vi "CRYGet Graph Name From Graph Type.vi"(11 "Graph Type":string) -> (2 "Type":enum16{"Curves", "Values", "Results", "WFM"}(ring), 3 "Graph Name":string)   [LabVIEW 2013]
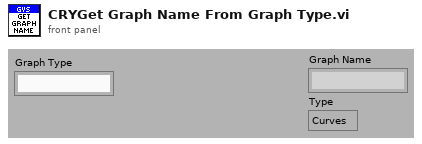
[diagram p1: front panel]
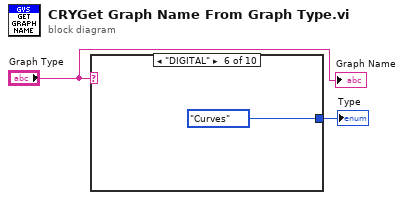
[diagram p0: block diagram]
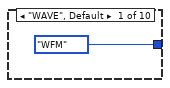
[diagram p2: hidden frame]
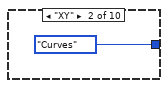
[diagram p3: hidden frame]
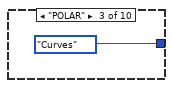
[diagram p4: hidden frame]
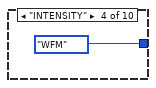
[diagram p5: hidden frame]
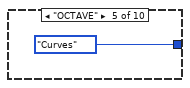
[diagram p6: hidden frame]
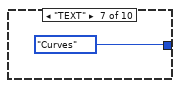
[diagram p7: hidden frame]
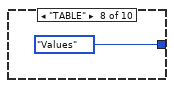
[diagram p8: hidden frame]
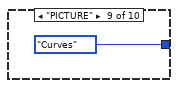
[diagram p9: hidden frame]
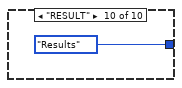
[diagram p10: hidden frame]
diagram:
  n1 = case shown="\"DIGITAL\"" "Graph Type" {
    tunnel: [enum16{"Curves", "Values", "Results", "WFM"}."WFM" ("Type") enum16{"Curves", "Values", "Results", "WFM"}."Curves" ("Type") enum16{"Curves", "Values", "Results", "WFM"}."Curves" ("Type") enum16{"Curves", "Values", "Results", "WFM"}."WFM" ("Type") enum16{"Curves", "Values", "Results", "WFM"}."Curves" ("Type") enum16{"Curves", "Values", "Results", "WFM"}."Curves" ("Type") enum16{"Curves", "Values", "Results", "WFM"}."Curves" ("Type") enum16{"Curves", "Values", "Results", "WFM"}."Values" ("Type") enum16{"Curves", "Values", "Results", "WFM"}."Curves" ("Type") enum16{"Curves", "Values", "Results", "WFM"}."Results" ("Type")] -> w2
    frame "WAVE", Default {
    }
    frame "XY" {
    }
    frame "POLAR" {
    }
    frame "INTENSITY" {
    }
    frame "OCTAVE" {
    }
    frame "DIGITAL" {
    }
    frame "TEXT" {
    }
    frame "TABLE" {
    }
    frame "PICTURE" {
    }
    frame "RESULT" {
    }
  }
  "Type" <- w2
  "Graph Name" <- "Graph Type"
